vi "Configure Multi Eval Meas List Range.vi"(7 "Number of Segments (1)":i32=1, 8 "error in (no error)":errorcluster, 9 "Start Index (1)":i32=1, 10 "Instance (1)":T1=1, 11 "VISA resource name":refnum<visa-resource-name>) -> (0 "error out":errorcluster, 3 "VISA resource name out":refnum<visa-resource-name>)   [LabVIEW 2015, in "Rohde&Schwarz CMXP NR FR2 Measurement.lvlib"]
doc: "Select a range of measured segments.\n\nAttribute:\nRSCMXPNRFR2M_ATTR_MULTI_EVAL_MEASUREMENT_LIST_RANGE\n\nRemote-control command:\nCONFigure:NRMMw:MEAS<i>:LIST:LRANge"
uses:
  <instrlib>/Rohde&Schwarz CMXP NR FR2 Measurement/Rohde&Schwarz CMXP NR FR2 Measurement.lvlib
  <instrlib>/Rohde&Schwarz CMXP NR FR2 Measurement/Private/_Instance.ctl
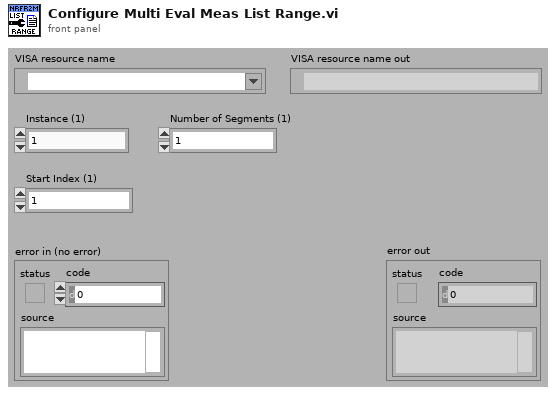
[diagram p1: front panel]
types:
  T1 = typedef "Rohde&Schwarz CMXP NR FR2 Measurement.lvlib/_Instance.ctl" = i32
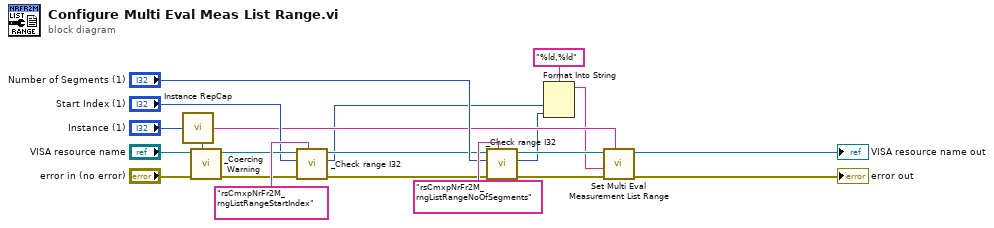
[diagram p0: block diagram]
diagram:
  n1 = call <instrlib>:"Instance RepCap.vi"("Instance In"="Instance (1)") -> ("In Range?"=w19:bool, "RepCap Identifier Out"=w9:string)  [unwired: 1 in]
  n2 = call <instrlib>:"_Coercing Warning.vi"("In Range?"=w19, "error in (no error)"="error in (no error)", "VISA resource name"="VISA resource name") -> ("error out"=w16:errorcluster, "VISA resource name out"=w17:refnum<visa-resource-name>)  [unwired: 7 in]
  n3 = call <instrlib>:"_Check range I32.vi"("Range Table Identifier"="rsCmxpNrFr2M_rngListRangeStartIndex", "error in (no error)"=w16, "I32 Value In"="Start Index (1)", "VISA resource name"=w17) -> ("error out"=w11:errorcluster, "I32 Value Out"=w4:i32, "VISA resource name out"=w12:refnum<visa-resource-name>)  [unwired: 5 in]
  n4 = call <instrlib>:"_Check range I32.vi"("Range Table Identifier"="rsCmxpNrFr2M_rngListRangeNoOfSegments", "error in (no error)"=w11, "I32 Value In"="Number of Segments (1)", "VISA resource name"=w12) -> ("error out"=w7:errorcluster, "I32 Value Out"=w3:i32, "VISA resource name out"=w8:refnum<visa-resource-name>)  [unwired: 5 in]
  n5 = Format Into String(format string="%ld,%ld", w4, w3) -> (resulting string=w1:string)  [unwired: 2 in, 1 out]
  n6 = call "Set Multi Eval Measurement List Range"("Repeated Capabilities"=w9, "error in (no error)"=w7, "Multi Eval Measurement List Range ()"=w1, "instrument handle"=w8) -> ("error out"=→"error out":errorcluster, "instrument handle out"=→"VISA resource name out":refnum<visa-resource-name>)  [unwired: 6 in]
